vi "STD校准画面.vi"() -> ()   [LabVIEW 2016, in "斯坦道原位多参数.lvlib"]
uses:
  <vilib>/Analysis/6fits.llb/Curve Fitting Criteria.ctl
  <vilib>/Plasmionique/MB Master/MB_Master_Serial/MB_Master_Serial.lvclass/MB_Master_Serial.ctl
  <vilib>/Plasmionique/MB Master/MB_Master_Serial/Read VISA Resource.vi
  <vilib>/Analysis/NI_AALPro.lvlib
  <vilib>/Plasmionique/MB Master/MB_VISA_Lock/MB_VISA_Lock.lvlib
  <vilib>/Plasmionique/MB Master/MB_Master_Serial/MB_Master_Serial.lvclass
panel:
  out "二次方程":cluster{"K":dbl, "B":dbl, "x^2":dbl} {"x^2" format="%#.6g"; "K" format="%#.6g"; "B" format="%#.6g"}
  out "r^2":dbl format="%.7f"
  out "拟合公式":string
  in  "精度":dbl=4.0
  in  "模型":enum32{"线性", "多项式", "折线"}(ring)
  out "XY图":cluster{"X Values":dbl[], "Y Values":dbl[]}[](graph)
  in  "第三点取值":bool
  in  "第二点取值":bool
  in  "第一点取值":bool
  out "实时信号值":sgl caption="信号值："
  out "实时检测值":sgl caption="检测值："
  in  "校准记录写入":bool
  in  "校准记录读取":bool
  in  "第三点信号值":sgl
  in  "第三点检测值":sgl
  in  "第三点标准值":sgl caption="第三点："
  in  "第二点信号值":sgl
  in  "第二点检测值":sgl
  in  "第二点标准值":sgl caption="第二点："
  in  "第一点信号值":sgl
  in  "第一点检测值":sgl
  in  "第一点标准值":sgl caption="第一点："
  out "传感器温度":sgl caption="传感器温度："
  in  "校准类型":u16(ring) caption="校准类型：" items=["单点校准"=1, "两点校准"=2, "三点校准"=3]
  out "校准时间":timestamp caption="校准时间：" format="%<%x %X>T"
  out "SN":string caption="探头序列号："
  in  "校准探头":u16(ring)=9 caption="校准探头：" items=["水温"=9, "pH值"=10, "溶解氧"=11, "电导率"=12, "浊度"=13, "叶绿素a"=14, "藻密度"=15, "氧化还原电位"=17, "溶解氧%"=18, "盐度"=19]
  # "探头校准"
  # "标准值"
  # "检测值"
  # "信号值"
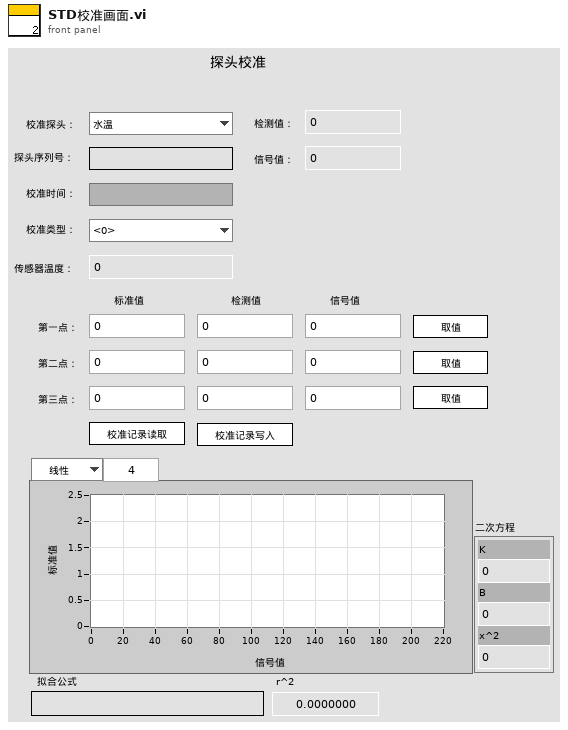
[diagram p1: front panel]
types:
  T1 = typedef "NI_AALPro.lvlib/Curve Fitting Criteria.ctl" = u16
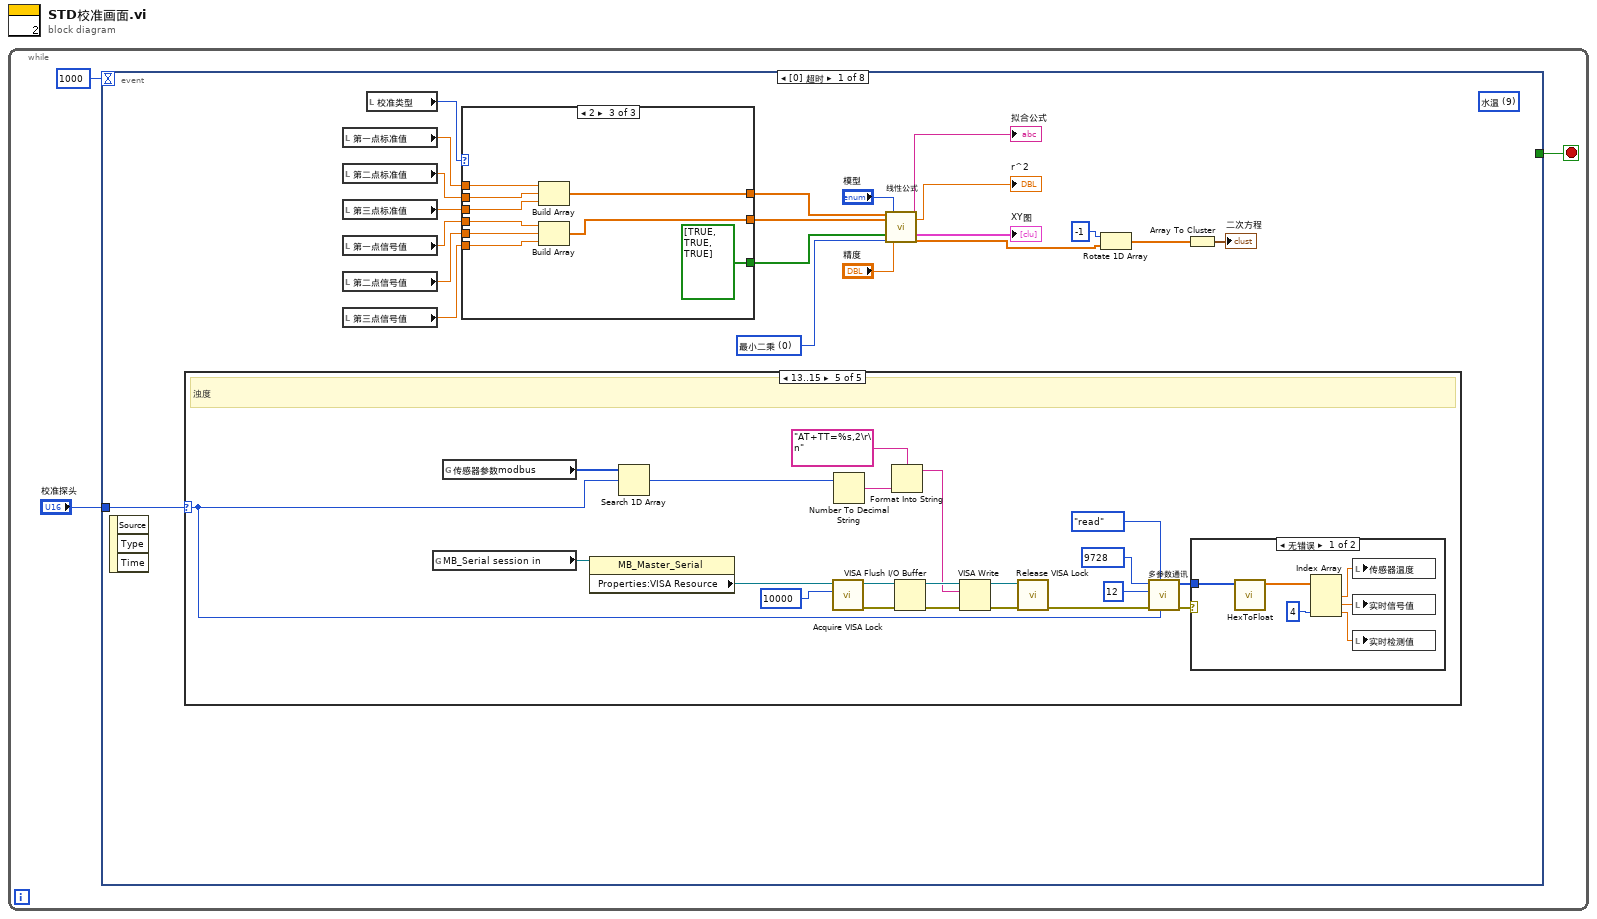
[diagram p0: block diagram]
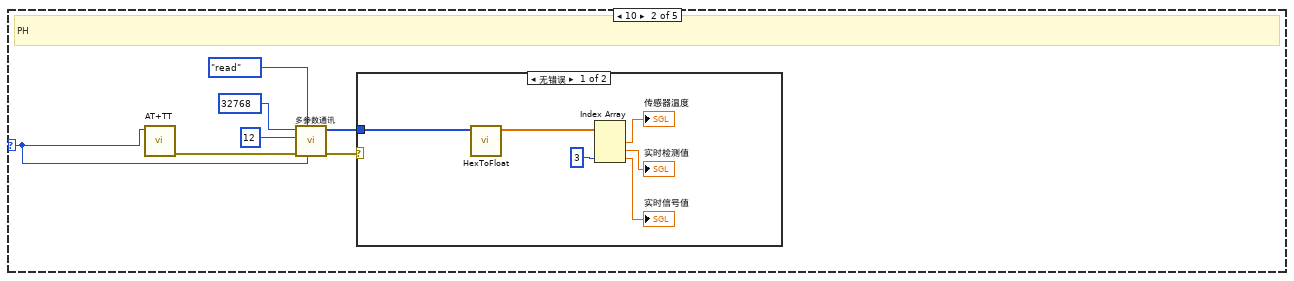
[diagram p3: hidden frame]
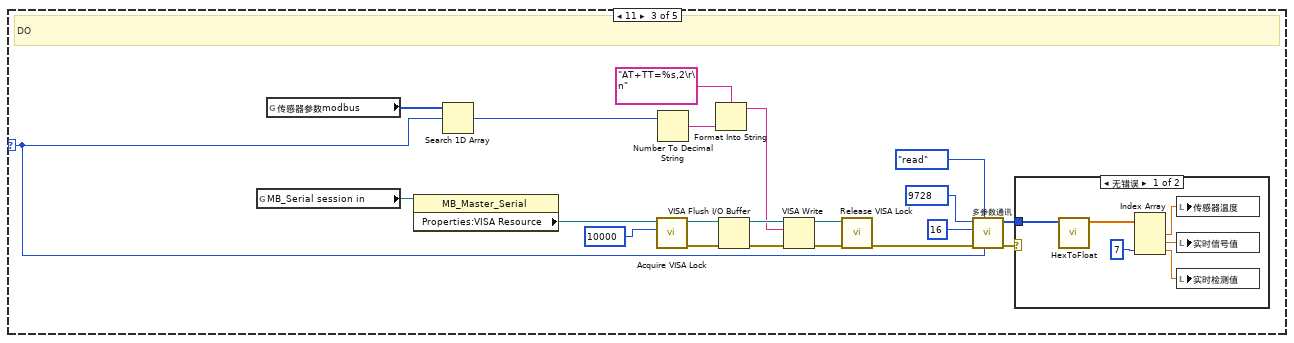
[diagram p5: hidden frame]
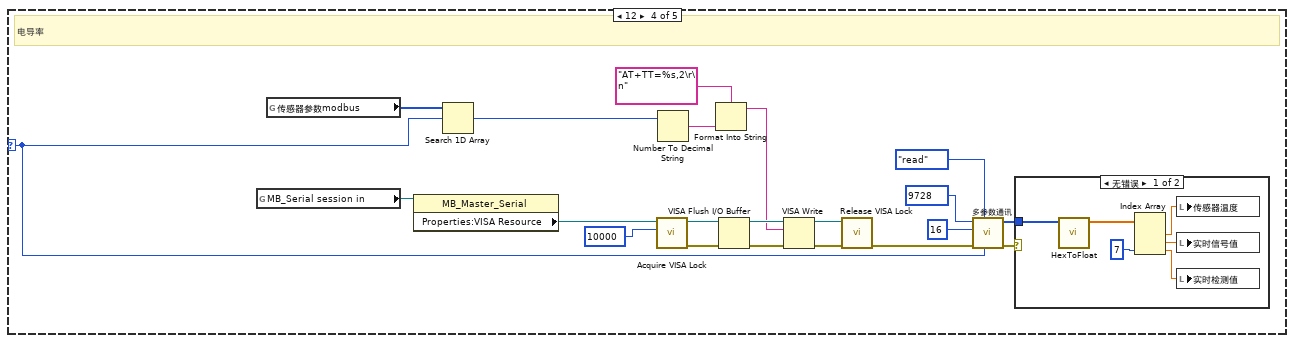
[diagram p7: hidden frame]
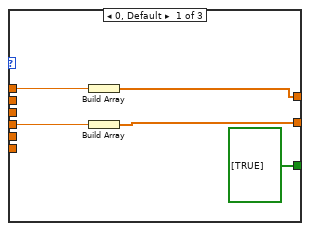
[diagram p10: hidden frame]
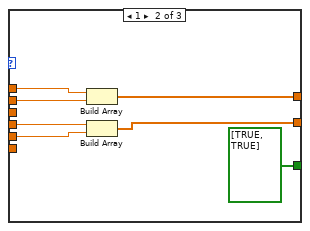
[diagram p11: hidden frame]
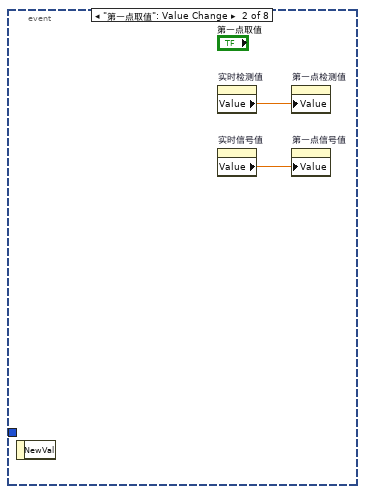
[diagram p12: hidden frame]
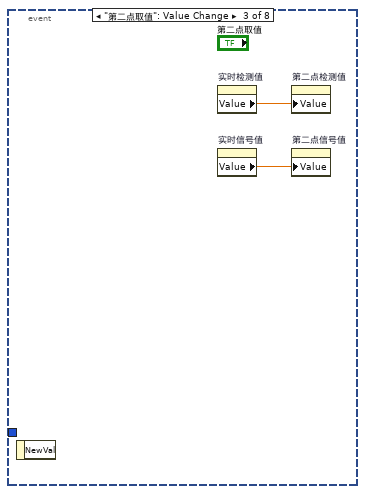
[diagram p13: hidden frame]
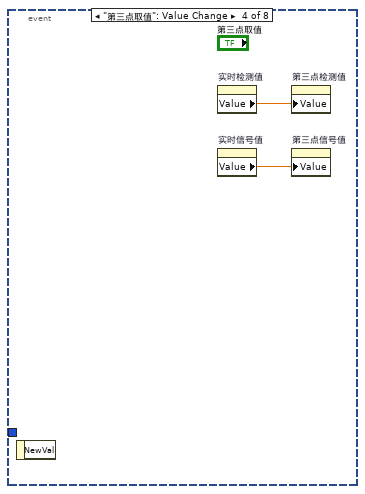
[diagram p14: hidden frame]
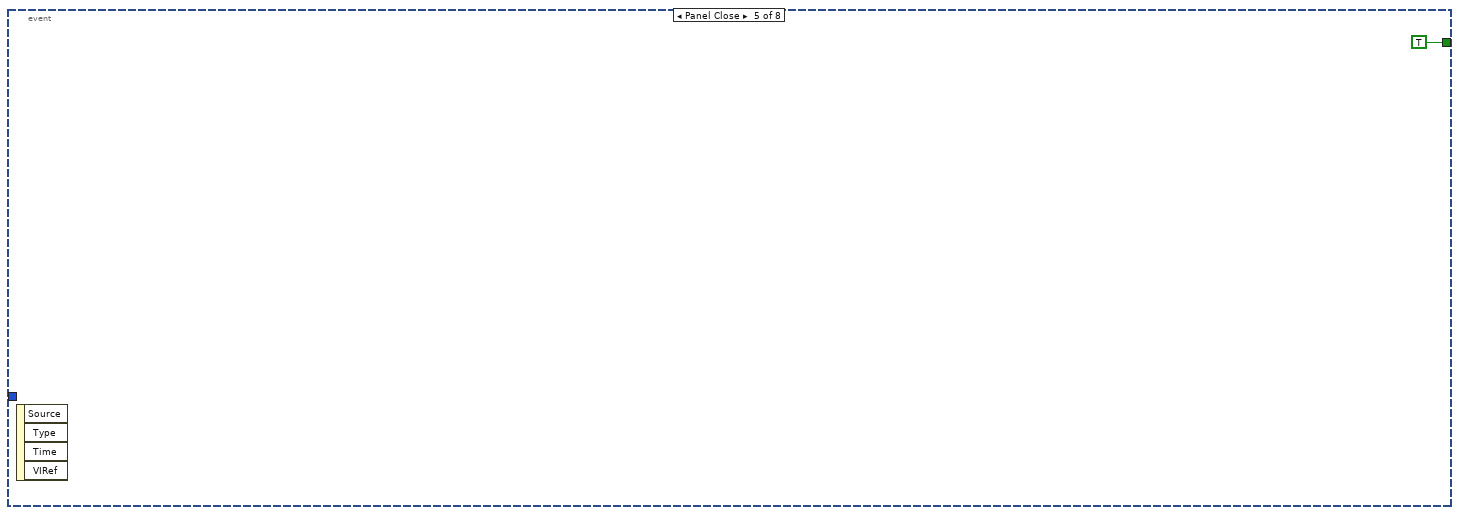
[diagram p15: hidden frame]
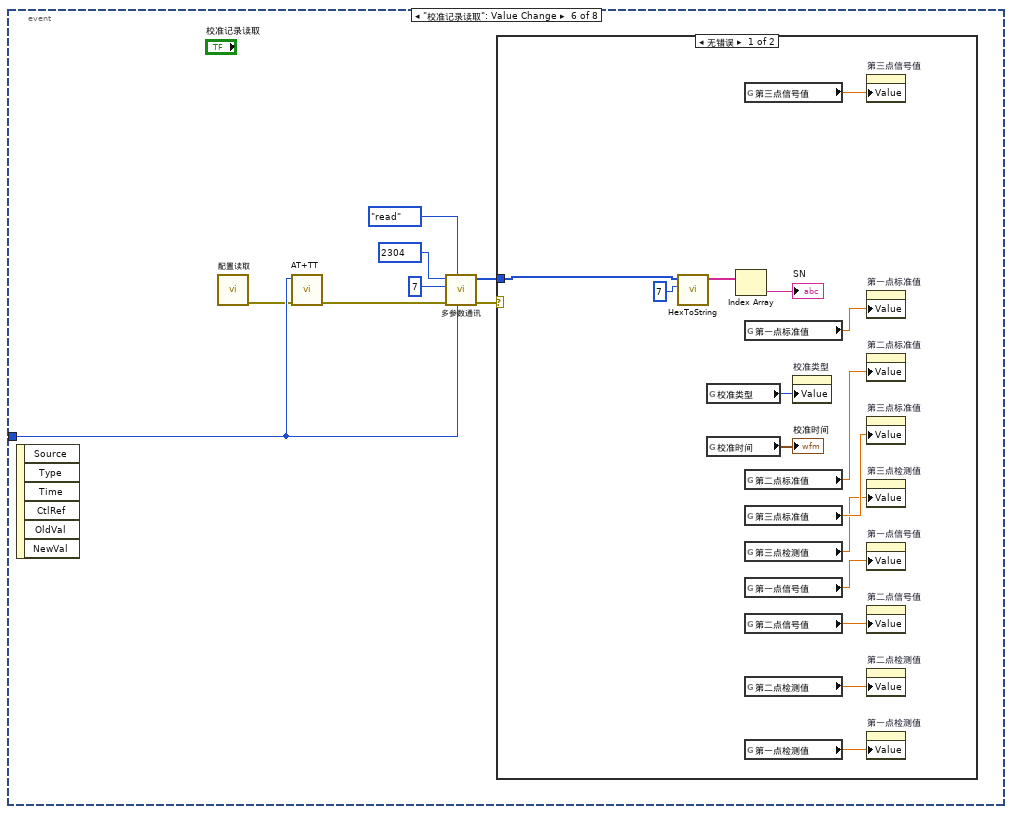
[diagram p16: hidden frame]
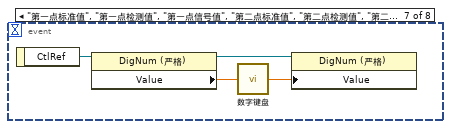
[diagram p18: hidden frame]
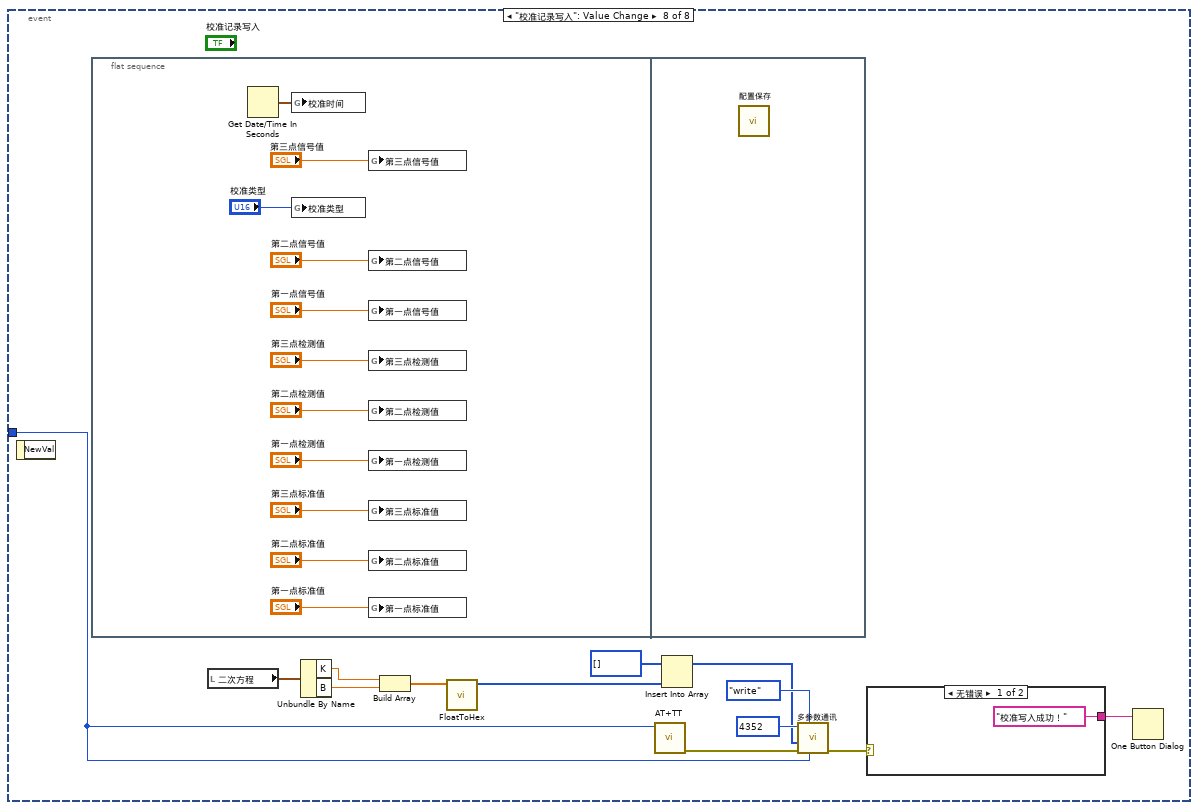
[diagram p19: hidden frame]
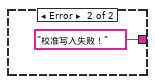
[diagram p20: hidden frame]
diagram:
  n1 = while {
    stop <- w3 stop-if-true
    n2 = event shown="[0] 超时" {
      selector: _ -> [_ _ _ _ _ _ _ _]
      dyn-events: _ -> [_ _ _ _ _ _ _ _]
      timeout: 1000 -> [_ _ _ _ _ _ _ _]
      tunnel: [_ _ _ _ TRUE _ _ _] -> w3
      tunnel: "校准探头" -> [w4 _ _ _ _ w150 _ w175]
      event Timeout {
        (unwired) u16 9 items=["水温"=9, "pH值"=10, "溶解氧"=11, "电导率"=12, "浊度"=13, "叶绿素a"=14, "藻密度"=15, "氧化还原电位"=17, "溶解氧%"=18, "盐度"=19] ("校准探头")
        w17 = T1 0 items=["最小二乘", "最小绝对残差", "Bisquare"] ("method")
        n3 = event-data() -> ()  [unwired: 1 in, 3 out]
        n4 = case shown="13..15" w4 {
          selector: w4 -> [_ w26 w39 w66 w93]
          frame 0, Default {
          }
          frame 10 {
            # "PH"
            n5 = call "AT+TT.vi"("站号"=w26) -> ("错误输出"=w25:errorcluster)  [unwired: 10 in]
            n6 = call "多参数通讯.vi"("Slave ID"=w26, "STEP"=enum16{"open", "read", "write", "close"}."read", "Error in"=w25, "quantity"=u16 12, "starting address"=u16 32768) -> ("error out"=w27:errorcluster, "Registers"=w31:u16[])  [unwired: 4 in, 1 out]
            n7 = case shown="无错误" w27 {
              tunnel: w31 -> [w36 _]
              frame No Error {
                n8 = call "HexToFloat.vi"("数组"=w36) -> ("FLOAT"=w37:sgl[])  [unwired: 10 in]
                n9 = Index Array(array=w37, index #3=3 ("索引")) -> (element #1=→"传感器温度":sgl, element #2=→"实时检测值":sgl, element #3=→"实时信号值":sgl)  [unwired: 2 in]
              }
              frame Error {
              }
            }
          }
          frame 11 {
            # "DO"
            n10 = global read "多参数全局变量.vi" "MB_Serial session in"() -> (w45:refnum<class "MB_Master_Serial.lvclass">)
            n11 = global read "多参数断电保存全局变量.vi" "传感器参数modbus"() -> (w43:u16[])
            n12 = property class="MB_Master_Serial"(reference=w45) -> ("Properties:VISA Resource"=w47:refnum<visa-resource-name>)  [unwired: 1 in, 2 out]
            n13 = Search 1D Array(1D array=w43, element=w39) -> (index of element=w42:i32)  [unwired: 1 in]
            n14 = call <vilib>:"Acquire VISA Lock.vi"("timeout in ms (-1)"=10000, "VISA resource name"=w47) -> ("error out"=w49:errorcluster, "VISA resource name out"=w48:refnum<visa-resource-name>)  [unwired: 8 in]
            n15 = Number To Decimal String(number=w42) -> (decimal integer string=w41:string)  [unwired: 1 in]
            n16 = Format Into String(format string="AT+TT=%s,2\r\n" ("写入缓冲区"), w41) -> (resulting string=w40:string)  [unwired: 2 in, 1 out]
            n17 = VISA Flush I/O Buffer(VISA resource name=w48, error in (no error)=w49) -> (VISA resource name out=w50:refnum<visa-resource-name>, error out=w51:errorcluster)  [unwired: 1 in]
            n18 = VISA Write(VISA resource name=w50, write buffer=w40, error in (no error)=w51) -> (VISA resource name out=w52:refnum<visa-resource-name>, error out=w53:errorcluster)  [unwired: 1 out]
            n19 = call <vilib>:"Release VISA Lock.vi"("error in (no error)"=w53, "VISA resource name"=w52) -> ("error out"=w38:errorcluster)  [unwired: 8 in, 1 out]
            n20 = call "多参数通讯.vi"("Slave ID"=w39, "STEP"=enum16{"open", "read", "write", "close"}."read", "Error in"=w38, "quantity"=u16 16, "starting address"=u16 9728) -> ("error out"=w54:errorcluster, "Registers"=w58:u16[])  [unwired: 4 in, 1 out]
            n21 = case shown="无错误" w54 {
              tunnel: w58 -> [w63 _]
              frame No Error {
                n22 = call "HexToFloat.vi"("数组"=w63) -> ("FLOAT"=w64:sgl[])  [unwired: 10 in]
                n23 = Index Array(array=w64, index #3=7 ("索引")) -> (element #1=w62:sgl, element #2=w61:sgl, element #3=w60:sgl)  [unwired: 2 in]
                n24 = local write "传感器温度"(w62) -> ()
                n25 = local write "实时信号值"(w61) -> ()
                n26 = local write "实时检测值"(w60) -> ()
              }
              frame Error {
              }
            }
          }
          frame 12 {
            # "电导率"
            n27 = global read "多参数全局变量.vi" "MB_Serial session in"() -> (w72:refnum<class "MB_Master_Serial.lvclass">)
            n28 = global read "多参数断电保存全局变量.vi" "传感器参数modbus"() -> (w70:u16[])
            n29 = property class="MB_Master_Serial"(reference=w72) -> ("Properties:VISA Resource"=w74:refnum<visa-resource-name>)  [unwired: 1 in, 2 out]
            n30 = Search 1D Array(1D array=w70, element=w66) -> (index of element=w69:i32)  [unwired: 1 in]
            n31 = call <vilib>:"Acquire VISA Lock.vi"("timeout in ms (-1)"=10000, "VISA resource name"=w74) -> ("error out"=w76:errorcluster, "VISA resource name out"=w75:refnum<visa-resource-name>)  [unwired: 8 in]
            n32 = Number To Decimal String(number=w69) -> (decimal integer string=w68:string)  [unwired: 1 in]
            n33 = Format Into String(format string="AT+TT=%s,2\r\n" ("写入缓冲区"), w68) -> (resulting string=w67:string)  [unwired: 2 in, 1 out]
            n34 = VISA Flush I/O Buffer(VISA resource name=w75, error in (no error)=w76) -> (VISA resource name out=w77:refnum<visa-resource-name>, error out=w78:errorcluster)  [unwired: 1 in]
            n35 = VISA Write(VISA resource name=w77, write buffer=w67, error in (no error)=w78) -> (VISA resource name out=w79:refnum<visa-resource-name>, error out=w80:errorcluster)  [unwired: 1 out]
            n36 = call <vilib>:"Release VISA Lock.vi"("error in (no error)"=w80, "VISA resource name"=w79) -> ("error out"=w65:errorcluster)  [unwired: 8 in, 1 out]
            n37 = call "多参数通讯.vi"("Slave ID"=w66, "STEP"=enum16{"open", "read", "write", "close"}."read", "Error in"=w65, "quantity"=u16 16, "starting address"=u16 9728) -> ("error out"=w81:errorcluster, "Registers"=w85:u16[])  [unwired: 4 in, 1 out]
            n38 = case shown="无错误" w81 {
              tunnel: w85 -> [w90 _]
              frame No Error {
                n39 = call "HexToFloat.vi"("数组"=w90) -> ("FLOAT"=w91:sgl[])  [unwired: 10 in]
                n40 = Index Array(array=w91, index #3=7 ("索引")) -> (element #1=w89:sgl, element #2=w88:sgl, element #3=w87:sgl)  [unwired: 2 in]
                n41 = local write "传感器温度"(w89) -> ()
                n42 = local write "实时信号值"(w88) -> ()
                n43 = local write "实时检测值"(w87) -> ()
              }
              frame Error {
              }
            }
          }
          frame 13..15 {
            # "浊度"
            n44 = global read "多参数全局变量.vi" "MB_Serial session in"() -> (w99:refnum<class "MB_Master_Serial.lvclass">)
            n45 = global read "多参数断电保存全局变量.vi" "传感器参数modbus"() -> (w97:u16[])
            n46 = property class="MB_Master_Serial"(reference=w99) -> ("Properties:VISA Resource"=w101:refnum<visa-resource-name>)  [unwired: 1 in, 2 out]
            n47 = Search 1D Array(1D array=w97, element=w93) -> (index of element=w96:i32)  [unwired: 1 in]
            n48 = call <vilib>:"Acquire VISA Lock.vi"("timeout in ms (-1)"=10000, "VISA resource name"=w101) -> ("error out"=w103:errorcluster, "VISA resource name out"=w102:refnum<visa-resource-name>)  [unwired: 8 in]
            n49 = Number To Decimal String(number=w96) -> (decimal integer string=w95:string)  [unwired: 1 in]
            n50 = Format Into String(format string="AT+TT=%s,2\r\n" ("写入缓冲区"), w95) -> (resulting string=w94:string)  [unwired: 2 in, 1 out]
            n51 = VISA Flush I/O Buffer(VISA resource name=w102, error in (no error)=w103) -> (VISA resource name out=w104:refnum<visa-resource-name>, error out=w105:errorcluster)  [unwired: 1 in]
            n52 = VISA Write(VISA resource name=w104, write buffer=w94, error in (no error)=w105) -> (VISA resource name out=w106:refnum<visa-resource-name>, error out=w107:errorcluster)  [unwired: 1 out]
            n53 = call <vilib>:"Release VISA Lock.vi"("error in (no error)"=w107, "VISA resource name"=w106) -> ("error out"=w92:errorcluster)  [unwired: 8 in, 1 out]
            n54 = call "多参数通讯.vi"("Slave ID"=w93, "STEP"=enum16{"open", "read", "write", "close"}."read", "Error in"=w92, "quantity"=u16 12, "starting address"=u16 9728) -> ("error out"=w108:errorcluster, "Registers"=w112:u16[])  [unwired: 4 in, 1 out]
            n55 = case shown="无错误" w108 {
              tunnel: w112 -> [w117 _]
              frame No Error {
                n56 = call "HexToFloat.vi"("数组"=w117) -> ("FLOAT"=w118:sgl[])  [unwired: 10 in]
                n57 = Index Array(array=w118, index #3=4 ("索引")) -> (element #1=w116:sgl, element #2=w115:sgl, element #3=w114:sgl)  [unwired: 2 in]
                n58 = local write "传感器温度"(w116) -> ()
                n59 = local write "实时信号值"(w115) -> ()
                n60 = local write "实时检测值"(w114) -> ()
              }
              frame Error {
              }
            }
          }
        }
        n61 = local read "第一点标准值"() -> (w22:sgl)
        n62 = local read "第二点标准值"() -> (w12:sgl)
        n63 = local read "第三点标准值"() -> (w10:sgl)
        n64 = local read "第一点信号值"() -> (w20:sgl)
        n65 = local read "第二点信号值"() -> (w11:sgl)
        n66 = local read "第三点信号值"() -> (w9:sgl)
        n67 = local read "校准类型"() -> (w24:u16)
        n68 = case shown="2" w24 {
          tunnel: [bool[] [TRUE] ("启用") bool[] [TRUE, TRUE] ("启用") bool[] [TRUE, TRUE, TRUE] ("启用")] -> w23
          tunnel: w22 -> [w122 w129 w138]
          tunnel: [w121 w127 w131] -> w21
          tunnel: w20 -> [w120 w126 w135]
          tunnel: [w119 w124 w132] -> w19
          tunnel: w12 -> [_ w128 w137]
          tunnel: w11 -> [_ w125 w134]
          tunnel: w10 -> [_ _ w136]
          tunnel: w9 -> [_ _ w133]
          frame 0, Default {
            n69 = Build Array(w122) -> (w121:sgl[])
            n70 = Build Array(w120) -> (w119:sgl[])
          }
          frame 1 {
            n71 = Build Array(w129, w128) -> (w127:sgl[])
            n72 = Build Array(w126, w125) -> (w124:sgl[])
          }
          frame 2 {
            n73 = Build Array(w138, w137, w136) -> (w131:sgl[])
            n74 = Build Array(w135, w134, w133) -> (w132:sgl[])
          }
        }
        n75 = call "线性公式.vi"("标液浓度"=w21, "信号值"=w19, "启用"=w23, "method"=w17, "模型"="模型", "精度"="精度") -> ("拟合方程"=→"拟合公式":string, "r^2"=→"r^2":dbl, "XY图"=→"XY图":cluster{"X Values":dbl[], "Y Values":dbl[]}[], "Polynomial Coefficients"=w6:dbl[])  [unwired: 7 in, 3 out]
        n76 = Rotate 1D Array(1:w6, 2:-1 ("n")) -> (0:w8:dbl[])
        n77 = Array To Cluster(array=w8) -> (cluster=→"二次方程":cluster{"[0]":dbl, "[1]":dbl, "[2]":dbl})
      }
      event "第一点取值": Value Change {
        n78 = event-data() -> ()  [unwired: 1 in, 1 out]
        n79 = property on="实时检测值" class="DigNum (严格)"() -> ("Value"=w141:sgl)  [unwired: 2 in, 2 out]
        n80 = property on="实时信号值" class="DigNum (严格)"() -> ("Value"=w140:sgl)  [unwired: 2 in, 2 out]
        n81 = property on="第一点检测值" class="DigNum (严格)"("Value"=w141) -> ()  [unwired: 2 in, 2 out]
        n82 = property on="第一点信号值" class="DigNum (严格)"("Value"=w140) -> ()  [unwired: 2 in, 2 out]
      }
      event "第二点取值": Value Change {
        n83 = event-data() -> ()  [unwired: 1 in, 1 out]
        n84 = property on="实时检测值" class="DigNum (严格)"() -> ("Value"=w143:sgl)  [unwired: 2 in, 2 out]
        n85 = property on="实时信号值" class="DigNum (严格)"() -> ("Value"=w142:sgl)  [unwired: 2 in, 2 out]
        n86 = property on="第二点检测值" class="DigNum (严格)"("Value"=w143) -> ()  [unwired: 2 in, 2 out]
        n87 = property on="第二点信号值" class="DigNum (严格)"("Value"=w142) -> ()  [unwired: 2 in, 2 out]
      }
      event "第三点取值": Value Change {
        n88 = event-data() -> ()  [unwired: 1 in, 1 out]
        n89 = property on="实时检测值" class="DigNum (严格)"() -> ("Value"=w145:sgl)  [unwired: 2 in, 2 out]
        n90 = property on="实时信号值" class="DigNum (严格)"() -> ("Value"=w144:sgl)  [unwired: 2 in, 2 out]
        n91 = property on="第三点检测值" class="DigNum (严格)"("Value"=w145) -> ()  [unwired: 2 in, 2 out]
        n92 = property on="第三点信号值" class="DigNum (严格)"("Value"=w144) -> ()  [unwired: 2 in, 2 out]
      }
      event Panel Close {
        n93 = event-data() -> ()  [unwired: 1 in, 4 out]
      }
      event "校准记录读取": Value Change {
        n94 = event-data() -> ()  [unwired: 1 in, 6 out]
        n95 = call "配置读取.vi"() -> ("error out"=w149:errorcluster)  [unwired: 11 in]
        n96 = call "AT+TT.vi"("错误输入（无错误）"=w149, "站号"=w150) -> ("错误输出"=w148:errorcluster)  [unwired: 9 in]
        n97 = call "多参数通讯.vi"("Slave ID"=w150, "STEP"=enum16{"open", "read", "write", "close"}."read", "Error in"=w148, "quantity"=u16 7, "starting address"=u16 2304) -> ("error out"=w147:errorcluster, "Registers"=w151:u16[])  [unwired: 4 in, 1 out]
        n98 = case shown="无错误" w147 {
          tunnel: w151 -> [w168 _]
          frame No Error {
            n99 = call "HexToString.vi"("字符个数"=7, "数组"=w168) -> ("STRING"=w169:string[])  [unwired: 9 in]
            n100 = global read "多参数断电保存全局变量.vi" "校准类型"() -> (w164:u16)
            n101 = global read "多参数断电保存全局变量.vi" "校准时间"() -> (→"校准时间":timestamp)
            n102 = Index Array(array=w169) -> (element=→"SN":string)  [unwired: 1 in]
            n103 = global read "多参数断电保存全局变量.vi" "第三点信号值"() -> (w157:sgl)
            n104 = global read "多参数断电保存全局变量.vi" "第一点标准值"() -> (w163:sgl)
            n105 = global read "多参数断电保存全局变量.vi" "第二点标准值"() -> (w162:sgl)
            n106 = global read "多参数断电保存全局变量.vi" "第三点标准值"() -> (w161:sgl)
            n107 = global read "多参数断电保存全局变量.vi" "第三点检测值"() -> (w160:sgl)
            n108 = global read "多参数断电保存全局变量.vi" "第一点信号值"() -> (w159:sgl)
            n109 = global read "多参数断电保存全局变量.vi" "第二点信号值"() -> (w158:sgl)
            n110 = global read "多参数断电保存全局变量.vi" "第二点检测值"() -> (w155:sgl)
            n111 = global read "多参数断电保存全局变量.vi" "第一点检测值"() -> (w156:sgl)
            n112 = property on="校准类型" class="Ring (严格)"("Value"=w164) -> ()  [unwired: 2 in, 2 out]
            n113 = property on="第三点信号值" class="DigNum (严格)"("Value"=w157) -> ()  [unwired: 2 in, 2 out]
            n114 = property on="第一点标准值" class="DigNum (严格)"("Value"=w163) -> ()  [unwired: 2 in, 2 out]
            n115 = property on="第二点标准值" class="DigNum (严格)"("Value"=w162) -> ()  [unwired: 2 in, 2 out]
            n116 = property on="第三点标准值" class="DigNum (严格)"("Value"=w161) -> ()  [unwired: 2 in, 2 out]
            n117 = property on="第三点检测值" class="DigNum (严格)"("Value"=w160) -> ()  [unwired: 2 in, 2 out]
            n118 = property on="第一点信号值" class="DigNum (严格)"("Value"=w159) -> ()  [unwired: 2 in, 2 out]
            n119 = property on="第二点信号值" class="DigNum (严格)"("Value"=w158) -> ()  [unwired: 2 in, 2 out]
            n120 = property on="第二点检测值" class="DigNum (严格)"("Value"=w155) -> ()  [unwired: 2 in, 2 out]
            n121 = property on="第一点检测值" class="DigNum (严格)"("Value"=w156) -> ()  [unwired: 2 in, 2 out]
          }
          frame Error {
          }
        }
      }
      event "第一点标准值", "第一点检测值", "第一点信号值", "第二点标准值", "第二点检测值", "第二点信号值", "第三点标准值", "第三点检测值", "第三点信号值": Mouse Down {
        n122 = event-data() -> ("CtlRef"=w173:refnum<vi>)  [unwired: 1 in]
        n123 = property class="DigNum (严格)"(reference=w173) -> (reference out=w170:refnum<vi>, "Value"=w172:sgl)  [unwired: 1 in, 1 out]
        n124 = call "数字键盘.vi"("OldNumber"=w172) -> ("NewNumber"=w171:dbl)
        n125 = property class="DigNum (严格)"(reference=w170, "Value"=w171) -> ()  [unwired: 1 in, 2 out]
      }
      event "校准记录写入": Value Change {
        n126 = event-data() -> ()  [unwired: 1 in, 1 out]
        n127 = flat-sequence {
          frame #0 {
            n128 = Get Date/Time In Seconds() -> (seconds since 1Jan1904=w188:timestamp)
            n129 = global write "多参数断电保存全局变量.vi" "校准时间"(w188) -> ()
            n130 = global write "多参数断电保存全局变量.vi" "校准类型"("校准类型") -> ()
            n131 = global write "多参数断电保存全局变量.vi" "第三点信号值"("第三点信号值") -> ()
            n132 = global write "多参数断电保存全局变量.vi" "第二点信号值"("第二点信号值") -> ()
            n133 = global write "多参数断电保存全局变量.vi" "第一点信号值"("第一点信号值") -> ()
            n134 = global write "多参数断电保存全局变量.vi" "第三点检测值"("第三点检测值") -> ()
            n135 = global write "多参数断电保存全局变量.vi" "第二点检测值"("第二点检测值") -> ()
            n136 = global write "多参数断电保存全局变量.vi" "第一点检测值"("第一点检测值") -> ()
            n137 = global write "多参数断电保存全局变量.vi" "第三点标准值"("第三点标准值") -> ()
            n138 = global write "多参数断电保存全局变量.vi" "第二点标准值"("第二点标准值") -> ()
            n139 = global write "多参数断电保存全局变量.vi" "第一点标准值"("第一点标准值") -> ()
          }
          frame #1 {
            n140 = call "配置保存.vi"() -> ()  [unwired: 11 in, 1 out]
          }
        }
        n141 = local read "二次方程"() -> (w179:cluster{"K":dbl, "B":dbl, "x^2":dbl})
        n142 = Unbundle By Name(w179) -> ("K"=w178:dbl, "B"=w177:dbl)
        n143 = Build Array(w178, w177) -> (w176:dbl[])
        n144 = call "FloatToHex.vi"("浮点数"=w176) -> ("DCBA整形输出"=w180:u16[])  [unwired: 10 in]
        n145 = call "AT+TT.vi"("站号"=w175) -> ("错误输出"=w174:errorcluster)  [unwired: 10 in]
        n146 = Insert Into Array(array=u16[] [] ("数组"), new element=w180) -> (w183:u16[])  [unwired: 1 in]
        n147 = call "多参数通讯.vi"("Slave ID"=w175, "STEP"=enum16{"open", "read", "write", "close"}."write", "Error in"=w174, "values"=w183, "starting address"=u16 4352) -> ("error out"=w182:errorcluster)  [unwired: 4 in, 2 out]
        n148 = case shown="无错误" w182 {
          tunnel: ["校准写入成功！" "校准写入失败！"] -> w186
          frame No Error {
          }
          frame Error {
          }
        }
        n149 = One Button Dialog(message=w186) -> ()  [unwired: 1 in, 1 out]
      }
    }
  }
